vi "ETH8_E2L_RTD2.vi"(10 "RTD 2 Off":dbl, 11 "Input Variable":dbl) -> (3 "RTD Value":dbl)   [LabVIEW 2022 SP3]
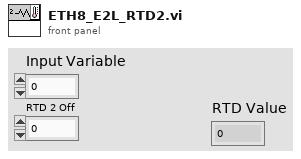
[diagram p1: front panel]
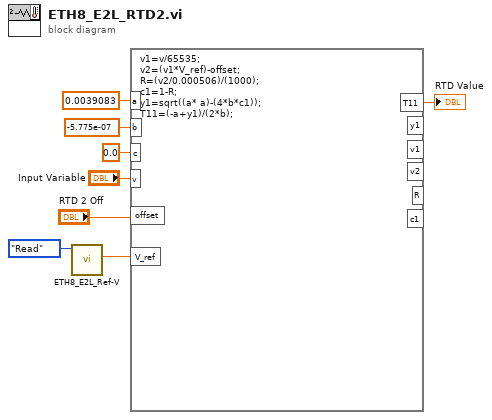
[diagram p0: block diagram]
diagram:
  n1 = call "ETH8_E2L_Ref-V.vi"("Write/Read"=enum16{"Write", "Read"}."Read") -> ("Ref voltage Out"=w1:dbl)  [unwired: 10 in]
  n2 = formula code="v1=v/65535;\nv2=(v1*V_ref)-offset;\nR=(v2/0.000506)/(1000);\nc1=1-R;\ny1=sqrt((a* a)-(4*b*c1));\nT11=(-a+y1)/(2*b);"("a"=0.0039083 ("input variable"), "b"=-5.775e-07 ("input variable"), "v"="Input Variable", "c"=0.0 ("input variable"), "offset"="RTD 2 Off", "V_ref"=w1) -> ("T11"=→"RTD Value":dbl)  [unwired: 5 out]
